vi "Register for Events.vi"(8 "error in (no error)":errorcluster, 11 "XY Stage Controller in":refnum<class "XY Stage Controller.lvclass">) -> (0 "error out":errorcluster, 2 "Event Refnums":T1, 3 "XY Stage Controller out":refnum<class "XY Stage Controller.lvclass">)   [LabVIEW 2022 SP3, in "XY Stage Controller.lvclass"]
uses:
  XY Stage Controller.lvclass
  XY Stage Data Class/XY Stage Data Class.lvclass
  Process Framework/Process State Data/Process State Data.lvclass
  XY Stage Data Class/XY Position.ctl
  XY Stage Data Class/Moving.ctl
  XY Stage Data Class/Homed.ctl
  XY Stage Data Class/Acceleration.ctl
  XY Stage Data Class/Current Speed.ctl
  XY Stage Data Class/Events.ctl
  Process Framework/Process State Data/Events.ctl
  XY Stage Data Class/Speed.ctl
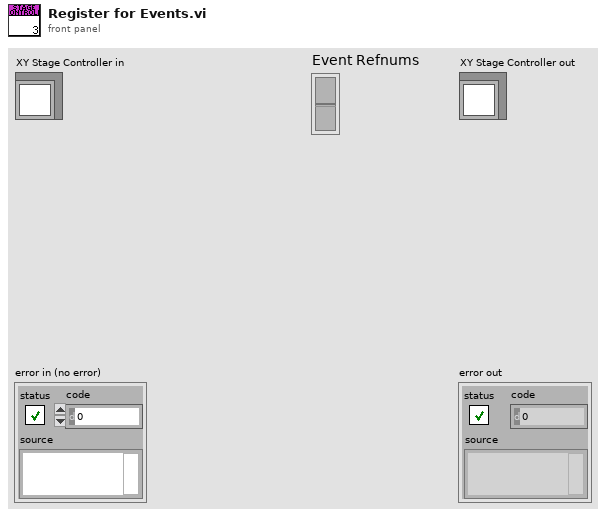
[diagram p1: front panel]
types:
  T1 = cluster{"Event Registration Refnum":refnum<event-registration>, "Event Registration Refnum":refnum<event-registration>}
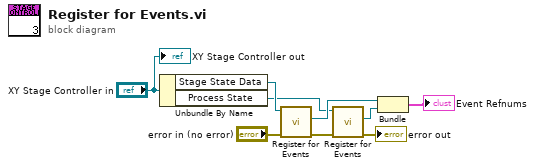
[diagram p0: block diagram]
diagram:
  n1 = Unbundle By Name("XY Stage Controller in") -> ("Stage State Data"=w8:refnum<data-value>, "Process State"=w5:refnum<data-value>)
  n2 = call "Register for Events.vi"("error in (no error)"="error in (no error)", "Stage State Data"=w8) -> ("error out"=w2:errorcluster, "Event Registration Refnum"=w6:refnum<event-registration>)  [unwired: 7 in, 1 out]
  n3 = call "Register for Events.vi"("error in (no error)"=w2, "Process State"=w5) -> ("error out"=→"error out":errorcluster, "Event Registration Refnum"=w4:refnum<event-registration>)  [unwired: 7 in, 1 out]
  n4 = Bundle("Event Registration Refnum"=w6, "Event Registration Refnum"=w4) -> (→"Event Refnums":T1)  [unwired: 1 in]
  "XY Stage Controller out" <- "XY Stage Controller in"
